vi "Find Actors.vi"(11 "Base Actor in":refnum<class "Base Actor.lvclass">) -> (2 "Actors":refnum<class "Actor.lvclass">[](array[class]))   [LabVIEW 2025, in "jettl.lvlib" / "Base Actor.lvlib" / "Base Actor.lvclass"]
uses:
  Base Actor.lvclass
  Actor/Actor.lvclass
  Base Actor.lvclass/Base Actor.ctl
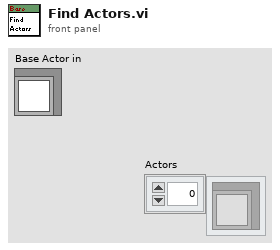
[diagram p1: front panel]
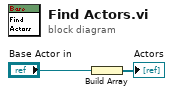
[diagram p0: block diagram]
diagram:
  n1 = Build Array("Base Actor in") -> (→"Actors":refnum<class "Base Actor.lvclass">[])
